vi "service_queue.vi"(8 "error in":errorcluster, 10 "queue in":refnum<queue>, 11 "connection ID":refnum<k5>) -> ()   [LabVIEW 2010]
uses:
  globals.vi
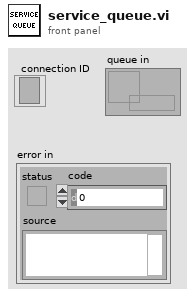
[diagram p1: front panel]
types:
  T1 = enum16{"Standard", "Buffered", "CRLF", "Immediate"}
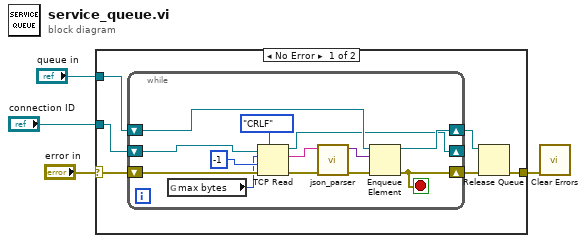
[diagram p0: block diagram]
diagram:
  n1 = case shown="No Error" "error in" {
    selector: "error in" -> [w5 w24]
    tunnel: "queue in" -> [w10 _]
    tunnel: "connection ID" -> [w9 _]
    tunnel: [w6 w24] -> w1
    frame No Error {
      n2 = while {
        shift-right: [w12] -> _
        shift-left: w9 -> [w21]
        shift-right: [w14] -> w7
        shift-left: w10 -> [w15]
        shift-right: [w16] -> w8
        shift-left: w5 -> [w13]
        stop <- w16 stop-if-true
        n3 = global read "globals.vi" "max bytes"() -> (w11:i32)
        n4 = TCP Read(connection ID=w21, bytes to read=w11, error in (no error)=w13, 7:T1."CRLF" ("mode (standard)"), 9:-1 ("timeout ms (25000)")) -> (connection ID out=w12:refnum<k5>, data out=w19:string, error out=w20:errorcluster)
        n5 = call "json_parser.vi"("error in"=w20, "JSON String"=w19) -> ("error out"=w18:errorcluster, "JSON Tree Out Passthrough"=w17:variant)  [unwired: 8 in]
        n6 = Enqueue Element(queue=w15, element=w17, error in (no error)=w18) -> (queue out=w14:refnum<queue>, error out=w16:errorcluster)  [unwired: 1 in, 1 out]
      }
      n7 = Release Queue(queue=w7, error in (no error)=w8) -> (error out=w6:errorcluster)  [unwired: 1 in, 2 out]
    }
    frame Error {
    }
  }
  n8 = call <vilib>:"Clear Errors.vi"("error in (no error)"=w1) -> ()  [unwired: 6 in, 1 out]
